vi "BarCodePrinting.vi"() -> ()   [LabVIEW 2010]
panel:
  out "error out":errorcluster
  in  "stop":bool
  in  "Data":string
  in  "Seagull_Drivers.ISDPrinter":refnum<k7>
  # "BarCode Data"
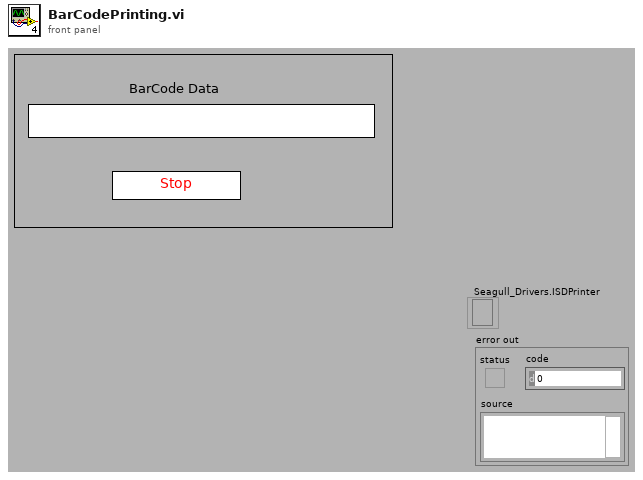
[diagram p1: front panel]
types:
  T1 = enum16{"open", "replace", "create", "open or create", "replace or create", "replace or create with confirmation"}
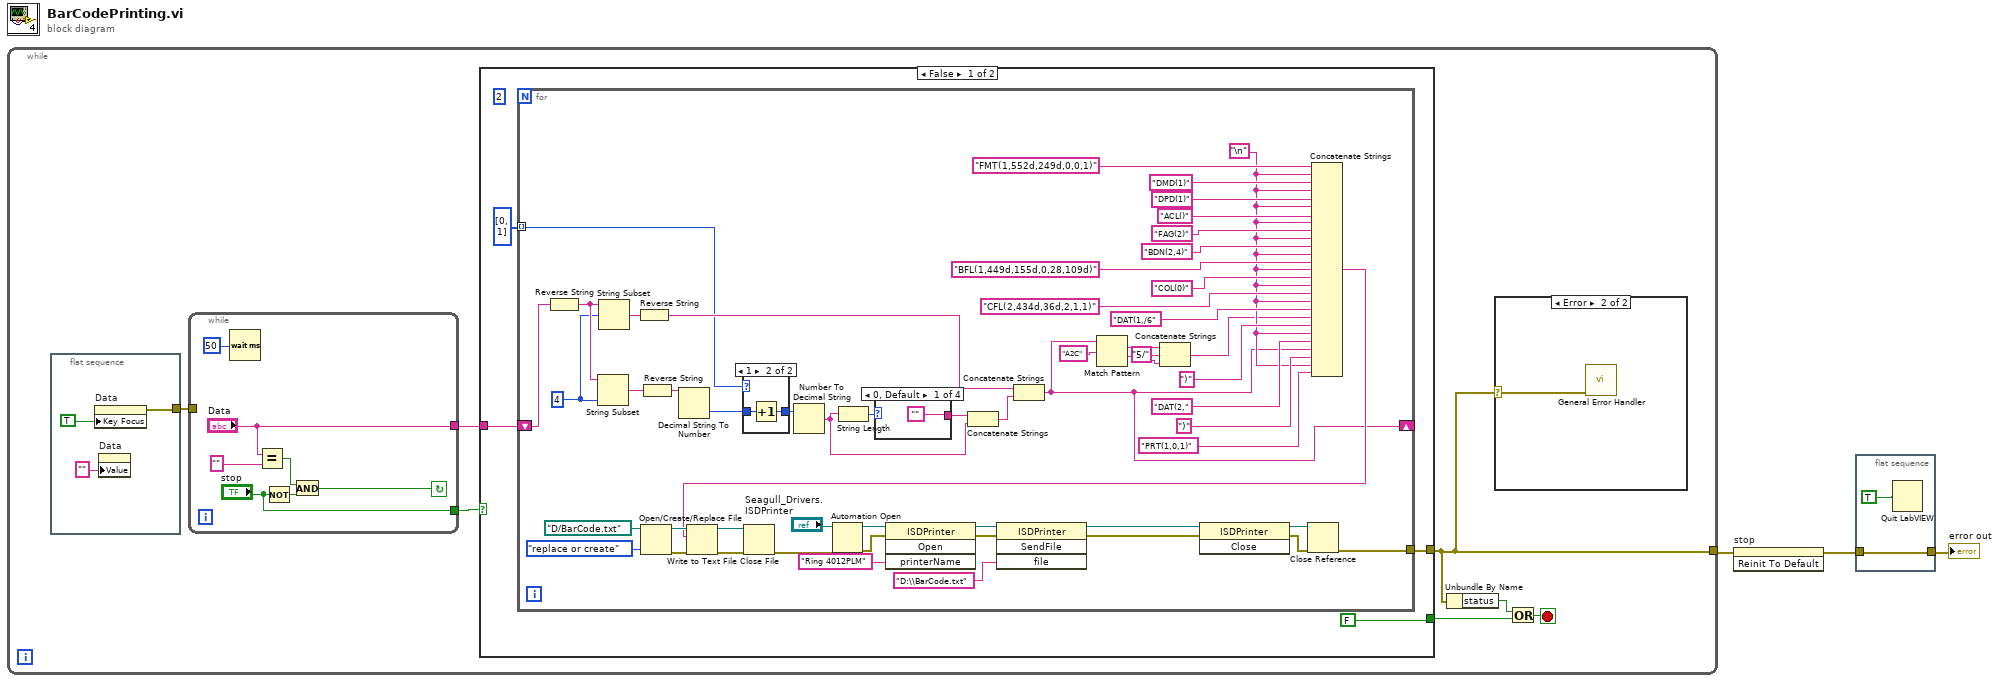
[diagram p0: block diagram]
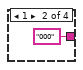
[diagram p4: hidden frame]
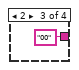
[diagram p5: hidden frame]
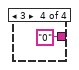
[diagram p6: hidden frame]
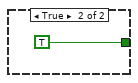
[diagram p7: hidden frame]
diagram:
  n1 = while {
    tunnel: [w4] -> w3
    stop <- w7 stop-if-true
    n2 = flat-sequence {
      tunnel: [w13] -> w8
      frame #0 {
        n3 = property on="Data" class="Str"("Key Focus"=TRUE) -> (error out=w13:errorcluster)  [unwired: 2 in, 1 out]
        n4 = property on="Data" class="Str"("Value"="" ("Data")) -> ()  [unwired: 2 in, 2 out]
      }
    }
    n5 = while {
      tunnel: ["Data"] -> w10
      tunnel: ["stop"] -> w9
      tunnel: w8 -> [_]
      stop <- w85 continue-if-true
      n6 = Wait (ms)(milliseconds to wait=u32 50) -> ()  [unwired: 1 out]
      n7 = Equal?(x="Data", y="") -> (x = y?=w82:bool)
      n8 = Not(x="stop") -> (.not. x?=w84:bool)
      n9 = And(x=w82, y=w84) -> (x .and. y?=w85:bool)
    }
    n10 = case shown="False" w9 {
      tunnel: w10 -> [w18 _]
      tunnel: [w17 _] -> w4
      tunnel: [FALSE ("Value") TRUE ("Value")] -> w5
      frame False {
        (unwired) 2
        n11 = for {
          tunnel: [w33] -> w17
          shift-right: [w23] -> _
          shift-left: w18 -> [w40]
          tunnel: i32[] [0, 1] -> [w25] mode=indexing
          w32 = 4 ("offset (0)")
          w44 = "\n"
          n12 = Reverse String(1:w40) -> (0:w35:string)
          n13 = String Subset(string=w35, length (rest)=w32) -> (substring=w36:string)  [unwired: 1 in]
          n14 = String Subset(string=w35, offset (0)=w32) -> (substring=w34:string)  [unwired: 1 in]
          n15 = Reverse String(1:w34) -> (0:w29:string)
          n16 = Open/Create/Replace File(file path (use dialog)=path "D:/BarCode.txt", operation (0:open)=T1."replace or create") -> (refnum out=w61:refnum<file>, error out=w41:errorcluster)  [unwired: 4 in, 1 out]
          n17 = Reverse String(1:w36) -> (0:w37:string)
          n18 = Decimal String To Number(string=w37) -> (number=w39:i32)  [unwired: 2 in, 1 out]
          n19 = case shown="1" w25 {
            tunnel: w39 -> [w74 w76]
            tunnel: [w74 w75] -> w38
            frame 0, Default {
            }
            frame 1 {
              n20 = Increment(x=w76) -> (x+1=w75:i32)
            }
          }
          n21 = Number To Decimal String(number=w38) -> (decimal integer string=w26:string)  [unwired: 1 in]
          n22 = String Length(string=w26) -> (length=w30:i32)
          n23 = case shown="0, Default" w30 {
            tunnel: ["" "000" ("string") "00" ("string") "0" ("string")] -> w27
            frame 0, Default {
            }
            frame 1 {
            }
            frame 2 {
            }
            frame 3 {
            }
          }
          n24 = Concatenate Strings(w27, w26) -> (w28:string)
          n25 = Concatenate Strings(w29, w28) -> (w23:string)
          n26 = Match Pattern(string=w23, regular expression="A2C") -> (match substring=w22:string, after substring=w20:string)  [unwired: 1 in, 2 out]
          n27 = Concatenate Strings(w22, "5/" ("string"), w20) -> (w19:string)
          n28 = Concatenate Strings("FMT(1,552d,249d,0,0,1)" ("string"), w44, "DMD(1)" ("string"), w44, "DPD(1)" ("string"), w44, "ACL()" ("string"), w44, "FAG(2)" ("string"), w44, "BDN(2,4)" ("string"), w44, "BFL(1,449d,155d,0,28,109d)" ("string"), w44, "COL(0)" ("string"), w44, "CFL(2,434d,36d,2,1,1)" ("string"), w44, "DAT(1,/6" ("string"), w19, ")" ("string"), w44, "DAT(2," ("string"), w23, ")" ("string"), w44, "PRT(1,0,1)" ("string")) -> (w42:string)
          n29 = Write to Text File(file (use dialog)=w61, text=w42, error in=w41) -> (refnum out=w59:refnum<file>, error out=w60:errorcluster)  [unwired: 1 in, 1 out]
          n30 = Close File(refnum=w59, error in=w60) -> (error out=w58:errorcluster)  [unwired: 1 out]
          n31 = Automation Open(error in (no error)=w58, Automation Refnum="Seagull_Drivers.ISDPrinter") -> (Automation Refnum=w67:refnum<k7>, error out=w68:errorcluster)  [unwired: 2 out]
          n32 = invoke class="ISDPrinter" method="Open"(reference=w67, error in=w68, "printerName"="Ring 4012PLM") -> (reference out=w71:refnum<k7>, error out=w69:errorcluster)  [unwired: 1 in, 2 out]
          n33 = invoke class="ISDPrinter" method="SendFile"(reference=w71, error in=w69, "file"="D:\\BarCode.txt" ("fileName")) -> (reference out=w65:refnum<k7>, error out=w64:errorcluster)  [unwired: 1 in, 2 out]
          n34 = invoke class="ISDPrinter" method="Close"(reference=w65, error in=w64) -> (reference out=w62:refnum<k7>, error out=w63:errorcluster)  [unwired: 1 in, 1 out]
          n35 = Close Reference(reference=w62, error in (no error)=w63) -> (error out=w33:errorcluster)
        }
      }
      frame True {
      }
    }
    n36 = Unbundle By Name(w4) -> ("status"=w6:bool)
    n37 = case shown="Error" w4 {
      selector: w4 -> [_ w11]
      frame No Error {
      }
      frame Error {
        n38 = call <vilib>:"General Error Handler.vi"("error in (no error)"=w11) -> ()  [unwired: 10 in, 5 out]
      }
    }
    n39 = Or(x=w6, y=w5) -> (x .or. y?=w7:bool)
  }
  n40 = invoke on="stop" class="Bool (strict)" method="Reinit To Default"(error in=w3) -> (error out=w2:errorcluster)  [unwired: 2 in, 2 out]
  n41 = flat-sequence {
    tunnel: w2 -> [w89]
    tunnel: [w89] -> w1
    frame #0 {
      n42 = Quit LabVIEW(quit? (T)=TRUE) -> ()
    }
  }
  "error out" <- w1
